vi "题目5.vi"() -> ()   [LabVIEW 2017]
panel:
  out "油量报警":bool
  in  "停止":bool
  in  "控制面板":T1 {"档位" scale=0.0..10.0; "油门" scale=0.0..10.0}
  out "显示面板":T2 {"油量" scale=0.0..200.0; "速度(km/h)" scale=0.0..300.0; "转速（r/s）" scale=0.0..8000.0}
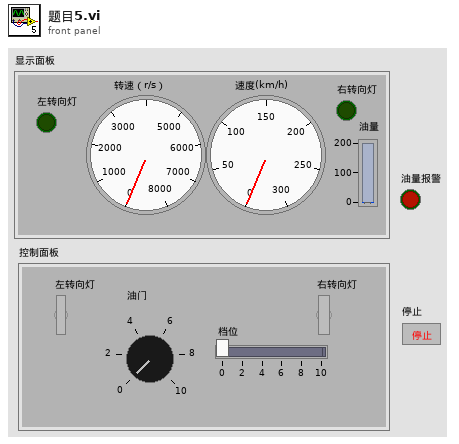
[diagram p1: front panel]
types:
  T1 = cluster{"左转向灯":bool, "油门":dbl, "档位":dbl, "右转向灯":bool}
  T2 = cluster{"左转向灯":bool, "右转向灯":bool, "转速（r/s）":dbl, "速度(km/h)":dbl, "油量":dbl}
  T3 = cluster{"左转向灯":bool, "右转向灯":bool, "油门":dbl, "档位":dbl, "y":dbl}
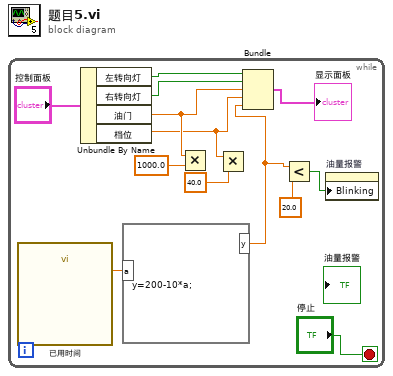
[diagram p0: block diagram]
diagram:
  n1 = while {
    stop <- "停止" stop-if-true
    n2 = call "已用时间"() -> ("Elapsed Time (s)"=w2:dbl)  [unwired: 12 in, 7 out]
    n3 = Unbundle By Name("控制面板") -> ("左转向灯"=w12:bool, "右转向灯"=w10:bool, "油门"=w8:dbl, "档位"=w6:dbl)
    n4 = formula code="y=200-10*a;"("a"=w2) -> ("y"=w4:dbl)
    n5 = Multiply(x=w8, y=1000.0) -> ()  [unwired: 1 out]
    n6 = Multiply(x=w6, y=40.0) -> ()  [unwired: 1 out]
    n7 = Bundle("左转向灯"=w12, "右转向灯"=w10, "油门"=w8, "档位"=w6, "y"=w4) -> (→"显示面板":T3)  [unwired: 1 in]
    n8 = Less?(x=w4, y=20.0) -> (x < y?=w1:bool)
    n9 = property on="油量报警" class="Bool (严格)"("Blinking"=w1) -> ()  [unwired: 2 in, 2 out]
  }
